vi "Get Results Path.vi"() -> (3 "Result Path":path=path "C:/PAS Circulation Tester")   [LabVIEW 2015]
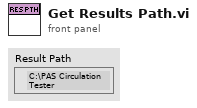
[diagram p1: front panel]
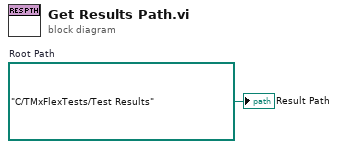
[diagram p0: block diagram]
diagram:
  w1 = path "C:/TMxFlexTests/Test Results"  # Root Path
  "Result Path" <- w1
